vi "KE622x -- Get Voltage Meas Units.vi"(0 "Resource In":refnum<visa-resource-name>, 1 "Check For SCPI Errors? (T)":bool=TRUE, 11 "error in (no error)":errorcluster) -> (4 "Resource Out (dupl)":refnum<visa-resource-name>, 8 "Voltage Meas Units":T1, 15 "error out":errorcluster)   [LabVIEW 2020, in "Keithley 622x.lvlib"]
doc: "Returns the units that will be returned for measurements (Ohms, Volts, Watts, or Siemens). It is assumed that a 2182/2182A is connected to the 6221 to perform the acutal measurementss (i.e. the 6221 has no measurement capability)."
uses:
  Keithley 622x.lvlib
  Typedefs/KE622x -- Voltage Meas Units.ctl
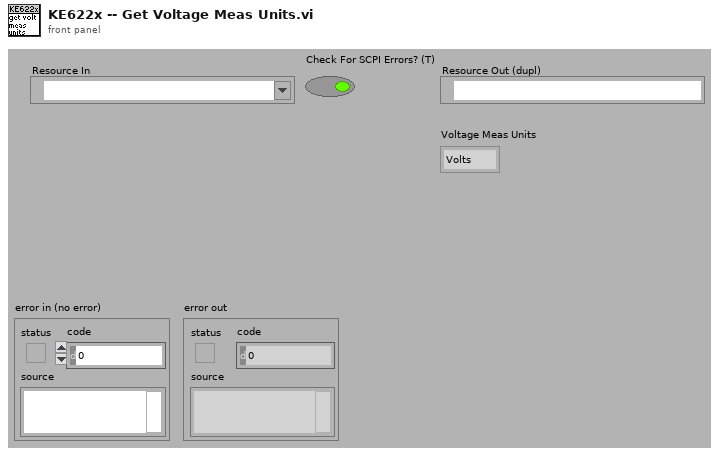
[diagram p1: front panel]
types:
  T1 = typedef "Keithley 622x.lvlib/KE622x -- Voltage Meas Units.ctl" = enum16{"Volts", "Ohms", "Watts", "Siemens"}
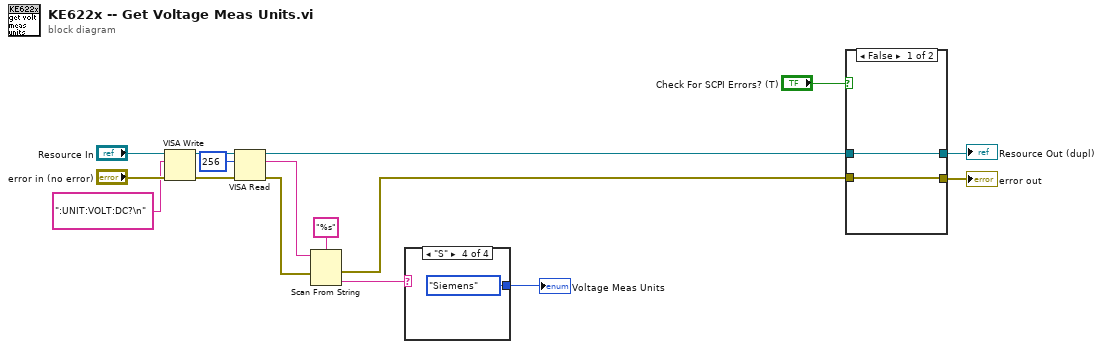
[diagram p0: block diagram]
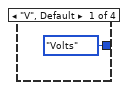
[diagram p2: hidden frame]
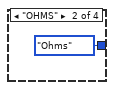
[diagram p3: hidden frame]
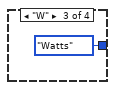
[diagram p4: hidden frame]
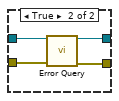
[diagram p5: hidden frame]
diagram:
  n1 = VISA Write(VISA resource name="Resource In", write buffer=":UNIT:VOLT:DC?\n" ("format string"), error in (no error)="error in (no error)") -> (VISA resource name out=w10:refnum<visa-resource-name>, error out=w9:errorcluster)  [unwired: 1 out]
  n2 = VISA Read(VISA resource name=w10, byte count=u32 256, error in (no error)=w9) -> (VISA resource name out=w7:refnum<visa-resource-name>, read buffer=w3:string, error out=w6:errorcluster)  [unwired: 1 out]
  n3 = Scan From String(format string="%s", input string=w3, error in=w6) -> (error out=w5:errorcluster, output 1=w2:string)  [unwired: 2 in, 2 out]
  n4 = case shown="\"S\"" w2 {
    tunnel: [KE622x_--_Voltage_Meas_Units."Volts" ("Voltage Meas Units") KE622x_--_Voltage_Meas_Units."Ohms" ("Voltage Meas Units") KE622x_--_Voltage_Meas_Units."Watts" ("Voltage Meas Units") KE622x_--_Voltage_Meas_Units."Siemens" ("Voltage Meas Units")] -> w1
    frame "V", Default {
    }
    frame "OHMS" {
    }
    frame "W" {
    }
    frame "S" {
    }
  }
  "Voltage Meas Units" <- w1
  n5 = case shown="False" "Check For SCPI Errors? (T)" {
    tunnel: w7 -> [w22 w26]
    tunnel: w5 -> [w21 w25]
    tunnel: [w21 w24] -> w12
    tunnel: [w22 w23] -> w13
    frame False {
    }
    frame True {
      n6 = call "Error Query.vi"("VISA Resource In"=w26, "error in (no error)"=w25) -> ("VISA Resource Out (dupl)"=w23:refnum<visa-resource-name>, "error out"=w24:errorcluster)  [unwired: 10 in, 2 out]
    }
  }
  "Resource Out (dupl)" <- w13
  "error out" <- w12
